vi "Read.vi"(8 "error in (no error)":errorcluster, 9 "timeout ms (25000)":i32, 10 "# bytes to read":i32, 11 "VISA TCP in":refnum<class "VISA TCP.lvclass">) -> (0 "error out":errorcluster, 2 "Read Bytes":u8[](array[numeric]), 3 "VISA TCP out":refnum<class "VISA TCP.lvclass">)   [LabVIEW 2013, in "Sockets.lvlib" / "VISA TCP.lvclass"]
doc: "Reads data from a socket connection."
uses:
  VISA TCP.lvclass
  VISA TCP.lvclass/VISA TCP.ctl
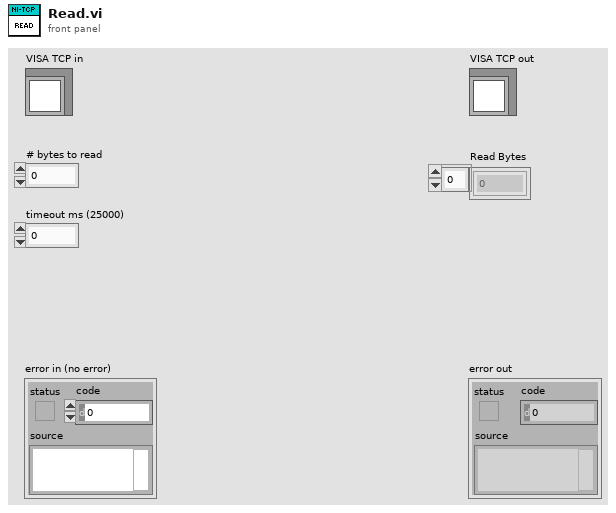
[diagram p1: front panel]
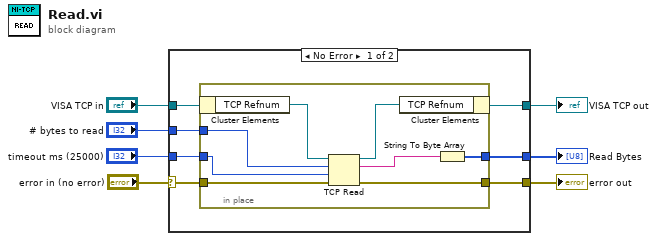
[diagram p0: block diagram]
diagram:
  n1 = case shown="No Error" "error in (no error)" {
    selector: "error in (no error)" -> [w8 w24]
    tunnel: "VISA TCP in" -> [w14 w23]
    tunnel: [w13 w23] -> w6
    tunnel: [w12 w24] -> w5
    tunnel: "timeout ms (25000)" -> [w11 _]
    tunnel: "# bytes to read" -> [w10 _]
    tunnel: [w9 _] -> w2
    frame No Error {
      n2 = in-place {
        in-place-border: w8 -> [w20]
        in-place-border: [w19] -> w12
        in-place-border: w10 -> [w18]
        in-place-border: w11 -> [w17]
        in-place-border: [w15] -> w9
        n3 = in-place-cluster #1(w14) -> ("TCP Refnum"=w22:refnum<k5>)
        n4 = TCP Read(connection ID=w22, bytes to read=w18, error in (no error)=w20, 9:w17) -> (connection ID out=w21:refnum<k5>, data out=w16:string, error out=w19:errorcluster)  [unwired: 1 in]
        n5 = in-place-cluster #1("TCP Refnum"=w21) -> (w13:refnum<class "VISA TCP.lvclass">)
        n6 = String To Byte Array(string=w16) -> (unsigned byte array=w15:u8[])
      }
    }
    frame Error {
    }
  }
  "error out" <- w5
  "VISA TCP out" <- w6
  "Read Bytes" <- w2
